vi "EOL CAN_Start CAN.vi"(8 "error in (no error)":errorcluster, 11 "CAN Interface":refnum<k21>="CAN1") -> (0 "error out":errorcluster, 1 "Tester Write Session out":refnum<k21>, 2 "Read Session out":refnum<k21>, 3 "DSC Write Session out":refnum<k21>, 5 "XNET Database":refnum<k21>)   [LabVIEW 2014]
uses:
  <vilib>/xnet/xnet.llb/XNET CAN Comm State.ctl
  <vilib>/xnet/xnet.llb/XNET Control Scope.ctl
  <vilib>/xnet/xnet.llb/XNET Frame CAN.ctl
  <vilib>/xnet/xnet.llb/XNET Frame Type CAN.ctl
  <vilib>/xnet/xnet.llb/XNET Create Session (Frame Input Queued).vi
  <vilib>/xnet/xnet.llb/XNET Create Session (Frame Output Single-point).vi
  <vilib>/xnet/xnet.llb/XNET Write (Frame CAN).vi
  <vilib>/xnet/xnet.llb/XNET Read (State CAN Comm).vi
  <vilib>/xnet/xnet.llb/XNET Wait (Interface Communicating).vi
  <resource>/objmgr/xnet.rc
panel:
  out "CAN:I/O Mode":u32(ring) items=["CAN 2.0", "CAN FD", "CAN FD+BRS"]
  out "Protocol":u32(ring) items=["CAN", "FlexRay", "LIN"]
  out "CAN:Transceiver Capability":u32(ring) items=["HS"=0, "LS"=1, "XS"=3, "XS (HS/LS)"=4]
  out "Interface:CAN:Transceiver State 3":u32(ring) items=["Normal", "Sleep", "Single Wire Wakeup", "Single Wire High-Speed"]
  out "Interface:CAN:Transceiver State 2":u32(ring) items=["Normal", "Sleep", "Single Wire Wakeup", "Single Wire High-Speed"]
  out "Interface:CAN:Transceiver State":u32(ring) items=["Normal", "Sleep", "Single Wire Wakeup", "Single Wire High-Speed"]
  out "PDUs":refnum<k21>[](array[refnum])
  out "Frames":refnum<k21>[](array[refnum])
  out "ECUs":refnum<k21>[](array[refnum])
  out "Database":refnum<k21>
  out "Configuration Status":i32
  out "CAN:Termination Capability":u32(ring) items=["No", "Yes"]
  out "Array":T1[](array[typedef]) items=["Error Active", "Error Passive", "Bus Off", "Init"]
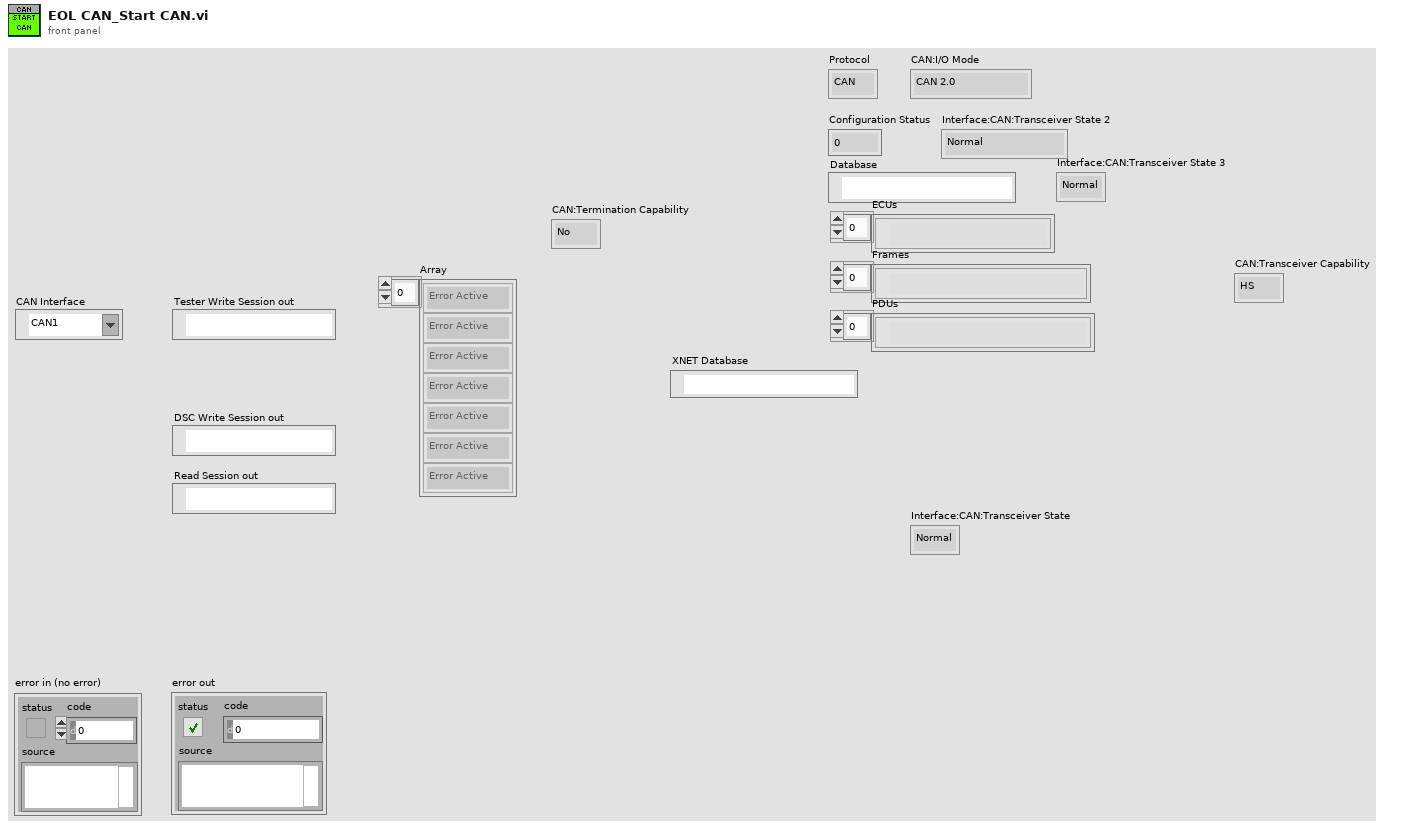
[diagram p1: front panel]
types:
  T1 = typedef "XNET CAN Comm State.ctl" = u8
  T2 = typedef "XNET Control Scope.ctl" = u32
  T3 = cluster{"Comment":string, "Default Payload":u8[], "Identifier":u32, "Name (Short)":string, "Payload Length":u32, "PDU_Mapping":cluster{"PDU":string, "Start Bit":u32, "Update Bit":i32}[], "CAN:Extended Identifier?":bool, "CAN:Timing Type":u32, "CAN:Transmit Time":dbl, "CAN:I/O Mode":u32}
  T4 = typedef "XNET Frame CAN.ctl" = cluster{"timestamp":timestamp, "payload":u8[], "identifier":u32, "type":T5, "extended?":bool, "echo?":bool}
  T5 = typedef "XNET Frame Type CAN.ctl" = u8
  T6 = typedef "XNET CAN Comm.ctl" = cluster{"fault code":i32, "fault?":bool, "communication state":T1, "last error":T7, "receive error counter":u8, "transmit error counter":u8, "transceiver error?":bool, "sleep?":bool}
  T7 = typedef "XNET CAN Last Err.ctl" = u8
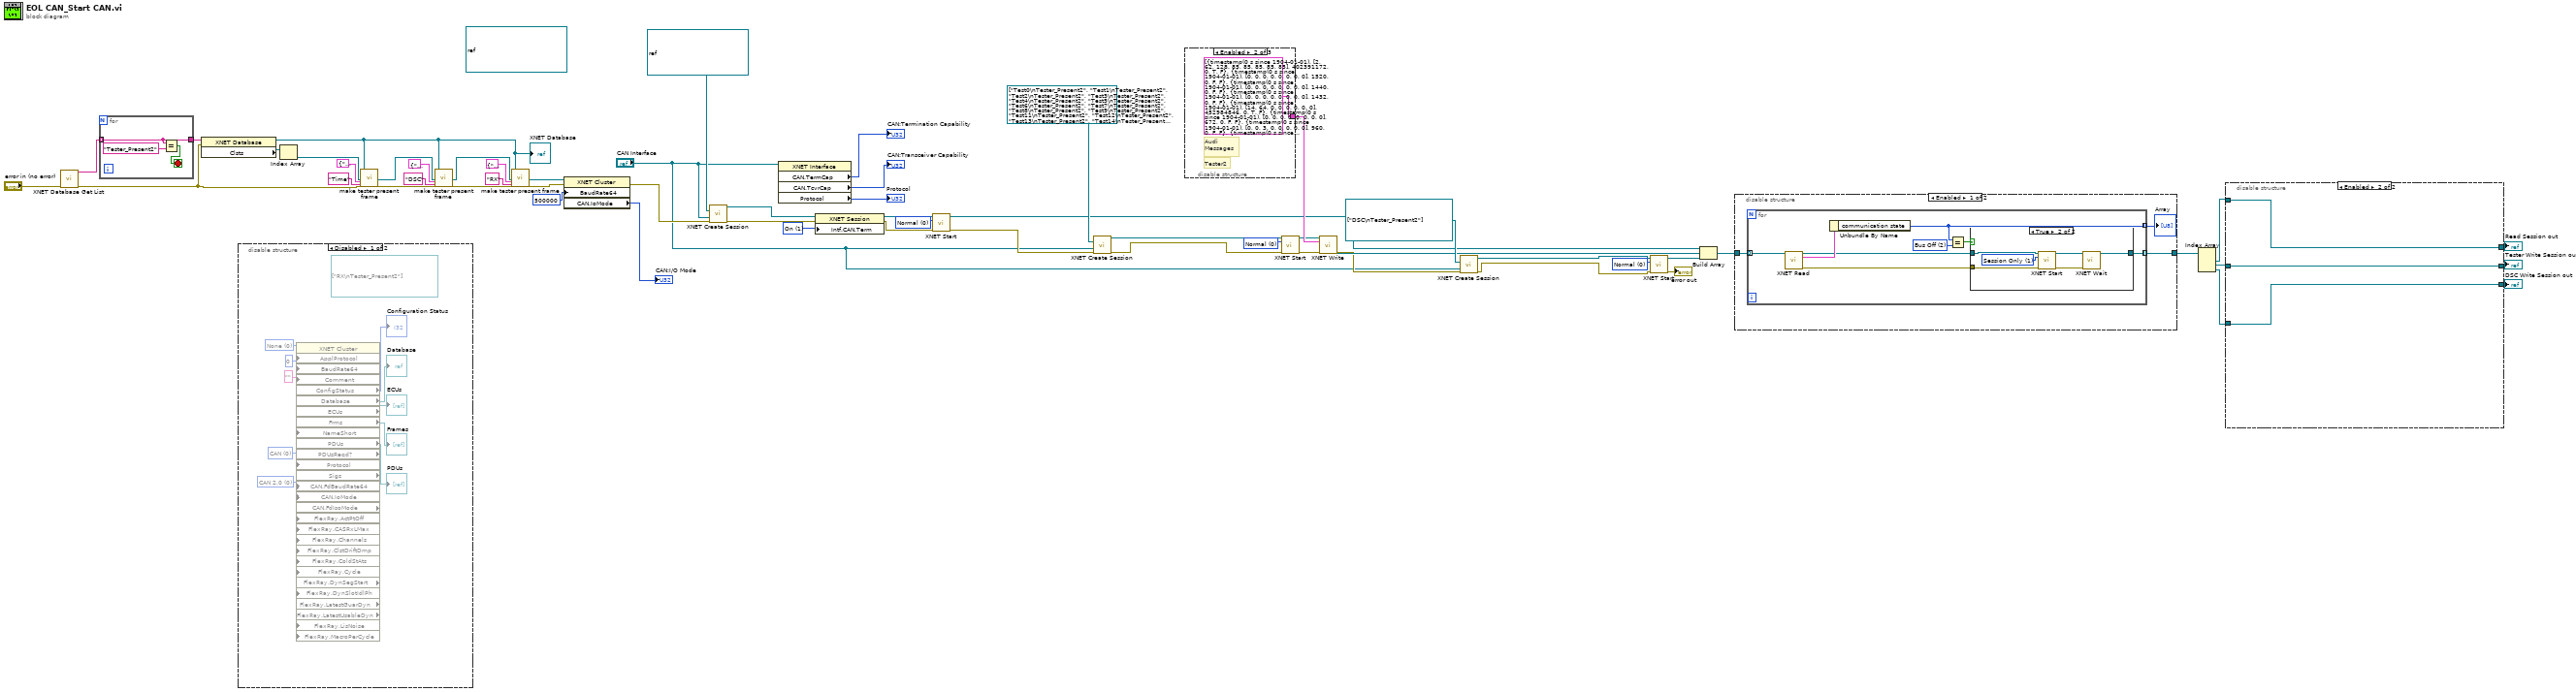
[diagram p0: block diagram]
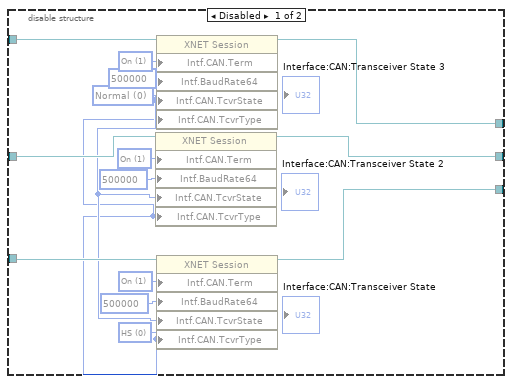
[diagram p3: hidden frame]
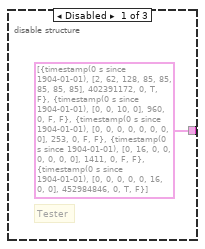
[diagram p6: hidden frame]
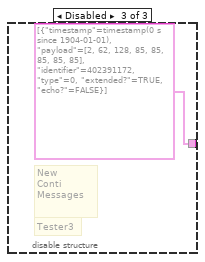
[diagram p7: hidden frame]
diagram:
  (unwired) refnum<k21> "RX\nTester_Present2" ("XNET Frame")
  w2 = u32 1 items=["Off", "On"] ("Interface:CAN:Termination")
  w22 = T2 0 items=["Normal", "Session Only", "Interface Only", "Session Only Blocking"] ("scope (normal)")
  w23 = T2 0 items=["Normal", "Session Only", "Interface Only", "Session Only Blocking"] ("scope (normal)")
  w24 = T2 0 items=["Normal", "Session Only", "Interface Only", "Session Only Blocking"] ("scope (normal)")
  n1 = call <vilib>:"XNET Database Get List.vi"("error in (no error)"="error in (no error)") -> ("array of alias"=w42:string[], "error out"=w38:errorcluster)  [unwired: 12 in, 1 out]
  n2 = for {
    tunnel: w42 -> [w59] mode=indexing
    tunnel: [w59] -> w41
    stop <- w60 stop-if-true
    n3 = Equal?(x=w59, y="Tester_Present2") -> (x = y?=w60:bool)
  }
  n4 = property class="XNET Database"(reference=w41, error in=w38) -> (reference out=w34:refnum<k21>, "Clsts"=w57:refnum<k21>[])  [unwired: 1 out]
  "XNET Database" <- w34
  n5 = disable-structure shown="Disabled" {
    frame Disabled {
      w62 = u32 0 items=["CAN 2.0", "CAN FD", "CAN FD+BRS"] ("CAN:I/O Mode")
      w63 = u32 0 items=["CAN", "FlexRay", "LIN"] ("Protocol")
      w71 = u32 0 items=["None", "J1939"] ("Application Protocol")
      (unwired) refnum<k21>[] ["RX\nTester_Present2"]
      n6 = property class="XNET Cluster" props=["ApplProtocol", "BaudRate64", "Comment", "ConfigStatus", "Database", "ECUs", "Frms", "NameShort", "PDUs", "PDUsReqd?", "Protocol", "Sigs", "CAN.FdBaudRate64", "CAN.IoMode", "CAN.FdIsoMode", "FlexRay.ActPtOff", "FlexRay.CASRxLMax", "FlexRay.Channels", "FlexRay.ClstDriftDmp", "FlexRay.ColdStAts", "FlexRay.Cycle", "FlexRay.DynSegStart", "FlexRay.DynSlotIdlPh", "FlexRay.LatestGuarDyn", "FlexRay.LatestUsableDyn", "FlexRay.LisNoise", "FlexRay.MacroPerCycle"]("ApplProtocol"=w71, "BaudRate64"=u64 0 ("64bit Baud Rate"), "Comment"="", "Protocol"=w63, "CAN.IoMode"=w62) -> ("ConfigStatus"=→"Configuration Status":i32, "Database"=→"Database":refnum<k21>, "ECUs"=→"ECUs":refnum<k21>[], "Frms"=→"Frames":refnum<k21>[], "PDUs"=→"PDUs":refnum<k21>[])  [unwired: 13 in, 8 out]
    }
    frame Enabled {
    }
  }
  n7 = Index Array(array=w57) -> (element=w36:refnum<k21>)  [unwired: 1 in]
  n8 = call "make tester present frame.vi"("Cluster::"=w36, "New Frame Properties"=T3 {"Comment"="DSC", "Default Payload"=[0, 0, 0, 0, 0, 0, 0, 0], "Identifier"=1714, "Name (Short)"="Time", "Payload Length"=8, "PDU_Mapping"=[], "CAN:Extended Identifier?"=FALSE, "CAN:Timing Type"=0, "CAN:Transmit Time"=0.001, "CAN:I/O Mode"=0}, "frame name"="Time", "error in (no error)"=w38, "database in"=w34) -> ("target cluster out"=w35:refnum<k21>, "error out"=w37:errorcluster)  [unwired: 21 in]
  n9 = call "make tester present frame.vi"("Cluster::"=w35, "New Frame Properties"=T3 {"Comment"="DSC", "Default Payload"=[0, 0, 0, 0, 0, 0, 0, 0], "Identifier"=402391172, "Name (Short)"="DSC", "Payload Length"=8, "PDU_Mapping"=[], "CAN:Extended Identifier?"=TRUE, "CAN:Timing Type"=1, "CAN:Transmit Time"=0.001, "CAN:I/O Mode"=0}, "frame name"="DSC", "error in (no error)"=w37, "database in"=w34) -> ("target cluster out"=w53:refnum<k21>, "error out"=w52:errorcluster)  [unwired: 21 in]
  n10 = call "make tester present frame.vi"("Cluster::"=w53, "New Frame Properties"=T3 {"Comment"="RX", "Default Payload"=[0, 127, 0, 0, 0, 0, 0, 0], "Identifier"=402522244, "Name (Short)"="RX", "Payload Length"=8, "PDU_Mapping"=[], "CAN:Extended Identifier?"=TRUE, "CAN:Timing Type"=1, "CAN:Transmit Time"=0.001, "CAN:I/O Mode"=0}, "frame name"="RX", "error in (no error)"=w52, "database in"=w34) -> ("target cluster out"=w44:refnum<k21>, "error out"=w43:errorcluster)  [unwired: 21 in]
  n11 = property class="XNET Cluster"(reference=w44, error in=w43, "BaudRate64"=u64 500000 ("64bit Baud Rate")) -> (error out=w56:errorcluster, "CAN.IoMode"=→"CAN:I/O Mode":u32)  [unwired: 1 out]
  n12 = call-poly <vilib>:"XNET Create Session.vi"("frame"=refnum<k21> "RX\nTester_Present2" ("XNET Frame"), "interface"="CAN Interface", "error in (no error)"=w56) -> ("session out"=w5:refnum<k21>, "error out"=w3:errorcluster)  [unwired: 11 in]
  n13 = property class="XNET Interface"(reference="CAN Interface") -> ("CAN.TermCap"=→"CAN:Termination Capability":u32, "CAN.TcvrCap"=→"CAN:Transceiver Capability":u32, "Protocol"=→"Protocol":u32)  [unwired: 1 in, 2 out]
  n14 = property class="XNET Session"(reference=w5, error in=w3, "Intf.CAN.Term"=w2) -> (reference out=w4:refnum<k21>, error out=w1:errorcluster)
  n15 = call <vilib>:"XNET Start.vi"("session in"=w4, "scope (normal)"=w24, "error in (no error)"=w1) -> ("session out"=w32:refnum<k21>, "error out"=w27:errorcluster)  [unwired: 11 in]
  n16 = call-poly <vilib>:"XNET Create Session.vi"("frame list"=refnum<k21>[] ["Test0\nTester_Present2", "Test1\nTester_Present2", "Test2\nTester_Present2", "Test3\nTester_Present2", "Test4\nTester_Present2", "Test5\nTester_Present2", "Test6\nTester_Present2", "Test7\nTester_Present2", "Test8\nTester_Present2", "Test9\nTester_Present2", "Test11\nTester_Present2", "Test12\nTester_Present2", "Test13\nTester_Present2", "Test14\nTester_Present2", "Test15\nTester_Present2", "Test16\nTester_Present2", "Test17\nTester_Present2", "Test18\nTester_Present2", "Test19\nTester_Present2", "Test20\nTester_Present2", "Test21\nTester_Present2", "Test22\nTester_Present2", "Test23\nTester_Present2", "Test24\nTester_Present2", "Test25\nTester_Present2", "Test26\nTester_Present2", "Test27\nTester_Present2"] ("Frames"), "interface"="CAN Interface", "error in (no error)"=w27) -> ("session out"=w19:refnum<k21>, "error out"=w20:errorcluster)  [unwired: 11 in]
  n17 = disable-structure shown="Enabled" {
    disable-tunnel: [T4[] [{"timestamp"=timestamp(0 s since 1904-01-01), "payload"=[2, 62, 128, 85, 85, 85, 85, 85], "identifier"=402391172, "type"=0, "extended?"=TRUE, "echo?"=FALSE}, {"timestamp"=timestamp(0 s since 1904-01-01), "payload"=[0, 0, 10, 0], "identifier"=960, "type"=0, "extended?"=FALSE, "echo?"=FALSE}, {"timestamp"=timestamp(0 s since 1904-01-01), "payload"=[0, 0, 0, 0, 0, 0, 0, 0], "identifier"=253, "type"=0, "extended?"=FALSE, "echo?"=FALSE}, {"timestamp"=timestamp(0 s since 1904-01-01), "payload"=[0, 16, 0, 0, 0, 0, 0, 0], "identifier"=1411, "type"=0, "extended?"=FALSE, "echo?"=FALSE}, {"timestamp"=timestamp(0 s since 1904-01-01), "payload"=[0, 0, 0, 0, 0, 16, 0, 0], "identifier"=452984846, "type"=0, "extended?"=TRUE, "echo?"=FALSE}] ("data") T4[] [{"timestamp"=timestamp(0 s since 1904-01-01), "payload"=[2, 62, 128, 85, 85, 85, 85, 85], "identifier"=402391172, "type"=0, "extended?"=TRUE, "echo?"=FALSE}, {"timestamp"=timestamp(0 s since 1904-01-01), "payload"=[0, 0, 0, 0, 0, 0, 0, 0], "identifier"=1520, "type"=0, "extended?"=FALSE, "echo?"=FALSE}, {"timestamp"=timestamp(0 s since 1904-01-01), "payload"=[0, 0, 0, 0, 0, 0, 0, 0], "identifier"=1440, "type"=0, "extended?"=FALSE, "echo?"=FALSE}, {"timestamp"=timestamp(0 s since 1904-01-01), "payload"=[0, 0, 0, 0, 0, 0, 0, 0], "identifier"=1432, "type"=0, "extended?"=FALSE, "echo?"=FALSE}, {"timestamp"=timestamp(0 s since 1904-01-01), "payload"=[14, 64, 0, 0, 0, 0, 0, 0], "identifier"=452984846, "type"=0, "extended?"=TRUE, "echo?"=FALSE}, {"timestamp"=timestamp(0 s since 1904-01-01), "payload"=[0, 0, 0, 0, 0, 0, 0, 0], "identifier"=672, "type"=0, "extended?"=FALSE, "echo?"=FALSE}, {"timestamp"=timestamp(0 s since 1904-01-01), "payload"=[0, 0, 3, 0, 0, 0, 0, 0], "identifier"=960, "type"=0, "extended?"=FALSE, "echo?"=FALSE}, {"timestamp"=timestamp(0 s since 1904-01-01), "payload"=[0, 0, 0, 0, 0, 0, 0, 0], "identifier"=1716, "type"=0, "extended?"=FALSE, "echo?"=FALSE}, {"timestamp"=timestamp(0 s since 1904-01-01), "payload"=[0, 16, 0, 0, 0, 0, 0, 0], "identifier"=1411, "type"=0, "extended?"=FALSE, "echo?"=FALSE}, {"timestamp"=timestamp(0 s since 1904-01-01), "payload"=[139, 64, 0, 0, 0, 0, 0, 0], "identifier"=452984971, "type"=0, "extended?"=TRUE, "echo?"=FALSE}, {"timestamp"=timestamp(0 s since 1904-01-01), "payload"=[0, 0, 0, 0, 0, 0, 0, 0], "identifier"=253, "type"=0, "extended?"=FALSE, "echo?"=FALSE}, {"timestamp"=timestamp(0 s since 1904-01-01), "payload"=[0, 0, 0, 0, 0, 0, 0, 0], "identifier"=508, "type"=0, "extended?"=FALSE, "echo?"=FALSE}, {"timestamp"=timestamp(0 s since 1904-01-01), "payload"=[0, 0, 0, 0, 150, 0, 0, 0], "identifier"=1646, "type"=0, "extended?"=FALSE, "echo?"=FALSE}, {"timestamp"=timestamp(0 s since 1904-01-01), "payload"=[0, 0, 0, 0, 0, 0, 0, 150], "identifier"=1719, "type"=0, "extended?"=FALSE, "echo?"=FALSE}, {"timestamp"=timestamp(0 s since 1904-01-01), "payload"=[0, 0, 4, 0, 0, 0, 0, 0], "identifier"=958, "type"=0, "extended?"=FALSE, "echo?"=FALSE}, {"timestamp"=timestamp(0 s since 1904-01-01), "payload"=[0, 0, 0, 0, 0, 0, 0, 0], "identifier"=1635, "type"=0, "extended?"=FALSE, "echo?"=FALSE}, {"timestamp"=timestamp(0 s since 1904-01-01), "payload"=[0, 0, 0, 0, 0, 0, 0, 0], "identifier"=319, "type"=0, "extended?"=FALSE, "echo?"=FALSE}, {"timestamp"=timestamp(0 s since 1904-01-01), "payload"=[0, 0, 0, 0, 0, 0, 0, 0], "identifier"=1616, "type"=0, "extended?"=FALSE, "echo?"=FALSE}, {"timestamp"=timestamp(0 s since 1904-01-01), "payload"=[0, 12, 0, 0, 0, 0, 0, 0], "identifier"=1413, "type"=0, "extended?"=FALSE, "echo?"=FALSE}, {"timestamp"=timestamp(0 s since 1904-01-01), "payload"=[0, 0, 0, 0, 0, 0, 0, 0], "identifier"=1462, "type"=0, "extended?"=FALSE, "echo?"=FALSE}, {"timestamp"=timestamp(0 s since 1904-01-01), "payload"=[16, 64, 0, 0, 0, 16, 0, 0], "identifier"=452984848, "type"=0, "extended?"=TRUE, "echo?"=FALSE}, {"timestamp"=timestamp(0 s since 1904-01-01), "payload"=[0, 0, 0, 0, 0, 0, 0, 0], "identifier"=976, "type"=0, "extended?"=FALSE, "echo?"=FALSE}, {"timestamp"=timestamp(0 s since 1904-01-01), "payload"=[0, 0, 0, 0, 0, 0, 0, 0], "identifier"=974, "type"=0, "extended?"=FALSE, "echo?"=FALSE}, {"timestamp"=timestamp(0 s since 1904-01-01), "payload"=[74, 64, 0, 0, 0, 0, 0, 0], "identifier"=452984906, "type"=0, "extended?"=TRUE, "echo?"=FALSE}, {"timestamp"=timestamp(0 s since 1904-01-01), "payload"=[0, 0, 0, 0, 0, 0, 0, 0], "identifier"=977, "type"=0, "extended?"=FALSE, "echo?"=FALSE}, {"timestamp"=timestamp(0 s since 1904-01-01), "payload"=[0, 0, 0, 0, 0, 0, 0, 0], "identifier"=975, "type"=0, "extended?"=FALSE, "echo?"=FALSE}, {"timestamp"=timestamp(0 s since 1904-01-01), "payload"=[75, 64, 0, 0, 0, 0, 0, 0], "identifier"=452984907, "type"=0, "extended?"=TRUE, "echo?"=FALSE}] ("Array 3") T4[] [{"timestamp"=timestamp(0 s since 1904-01-01), "payload"=[2, 62, 128, 85, 85, 85, 85, 85], "identifier"=402391172, "type"=0, "extended?"=TRUE, "echo?"=FALSE}] ("data")] -> w55
    frame Disabled {
      # "Tester"
    }
    frame Enabled {
      # "Tester2"
      # "Audi\nMessages"
    }
    frame Disabled {
      # "Tester3"
      # "New\nConti\nMessages"
    }
  }
  n18 = call <vilib>:"XNET Start.vi"("session in"=w19, "scope (normal)"=w23, "error in (no error)"=w20) -> ("session out"=w54:refnum<k21>, "error out"=w47:errorcluster)  [unwired: 11 in]
  n19 = call-poly <vilib>:"XNET Write.vi"("session in"=w54, "data"=w55, "error in (no error)"=w47) -> ("session out"=w31:refnum<k21>, "error out"=w26:errorcluster)  [unwired: 11 in]
  n20 = call-poly <vilib>:"XNET Create Session.vi"("frame list"=refnum<k21>[] ["DSC\nTester_Present2"] ("Frames"), "interface"="CAN Interface", "error in (no error)"=w26) -> ("session out"=w18:refnum<k21>, "error out"=w17:errorcluster)  [unwired: 11 in]
  n21 = call <vilib>:"XNET Start.vi"("session in"=w18, "scope (normal)"=w22, "error in (no error)"=w17) -> ("session out"=w30:refnum<k21>, "error out"=→"error out":errorcluster)  [unwired: 11 in]
  n22 = Build Array(w32, w31, w30) -> (w29:refnum<k21>[])
  n23 = disable-structure shown="Enabled" {
    disable-tunnel: w29 -> [w77 w93]
    disable-tunnel: [w75 w93] -> w28
    frame Enabled {
      n24 = for {
        tunnel: w77 -> [w84] mode=indexing
        tunnel: [w79] -> w76 mode=indexing
        tunnel: [w78] -> w75 mode=indexing
        w83 = T1 2 items=["Error Active", "Error Passive", "Bus Off", "Init"] ("y")
        n25 = call-poly <vilib>:"XNET Read.vi"("session in"=w84) -> ("session out"=w81:refnum<k21>, "CAN comm"=w85:T6, "error out"=w80:errorcluster)  [unwired: 12 in]
        n26 = Unbundle By Name(w85) -> ("communication state"=w79:T1)
        n27 = Equal?(x=w79, y=w83) -> (x = y?=w82:bool)
        n28 = case shown="True" w82 {
          tunnel: w81 -> [w86 w92]
          tunnel: w80 -> [_ w90]
          tunnel: [w86 w87] -> w78
          frame False {
          }
          frame True {
            w88 = T2 1 items=["Normal", "Session Only", "Interface Only", "Session Only Blocking"] ("scope (normal)")
            n29 = call <vilib>:"XNET Start.vi"("session in"=w92, "scope (normal)"=w88, "error in (no error)"=w90) -> ("session out"=w91:refnum<k21>, "error out"=w89:errorcluster)  [unwired: 11 in]
            n30 = call-poly <vilib>:"XNET Wait.vi"("session in"=w91, "error in (no error)"=w89) -> ("session out"=w87:refnum<k21>)  [unwired: 12 in, 1 out]
          }
        }
      }
      "Array" <- w76
    }
    frame Disabled {
    }
  }
  n31 = Index Array(array=w28) -> (element #1=w14:refnum<k21>, element #2=w12:refnum<k21>, element #3=w10:refnum<k21>)  [unwired: 3 in]
  n32 = disable-structure shown="Enabled" {
    disable-tunnel: w14 -> [w106 w110]
    disable-tunnel: [w105 w110] -> w13
    disable-tunnel: w12 -> [w102 w109]
    disable-tunnel: [w101 w109] -> w11
    disable-tunnel: w10 -> [w100 w108]
    disable-tunnel: [w99 w108] -> w9
    frame Disabled {
      w94 = u32 0 items=["HS", "LS", "SW", "Ext", "Disc"] ("Interface:CAN:Transceiver Type")
      w95 = u32 0 items=["Normal", "Sleep", "Single Wire Wakeup", "Single Wire High-Speed"] ("Interface:CAN:Transceiver State")
      w103 = u32 1 items=["Off", "On"] ("Interface:CAN:Termination")
      w104 = u32 1 items=["Off", "On"] ("Interface:CAN:Termination")
      w107 = u32 1 items=["Off", "On"] ("Interface:CAN:Termination")
      n33 = property class="XNET Session"(reference=w102, "Intf.CAN.Term"=w104, "Intf.BaudRate64"=u64 500000 ("Interface:64bit Baud Rate"), "Intf.CAN.TcvrState"=w95, "Intf.CAN.TcvrType"=w94) -> (reference out=w101:refnum<k21>)  [unwired: 1 in, 1 out]
      n34 = property class="XNET Session"(reference=w106, "Intf.CAN.Term"=w107, "Intf.BaudRate64"=u64 500000 ("Interface:64bit Baud Rate"), "Intf.CAN.TcvrState"=w95, "Intf.CAN.TcvrType"=w94) -> (reference out=w105:refnum<k21>)  [unwired: 1 in, 1 out]
      n35 = property class="XNET Session"(reference=w100, "Intf.CAN.Term"=w103, "Intf.BaudRate64"=u64 500000 ("Interface:64bit Baud Rate"), "Intf.CAN.TcvrState"=w95, "Intf.CAN.TcvrType"=w94) -> (reference out=w99:refnum<k21>)  [unwired: 1 in, 1 out]
    }
    frame Enabled {
    }
  }
  "Tester Write Session out" <- w11
  "Read Session out" <- w13
  "DSC Write Session out" <- w9
